vi "camera defaults globals - SubVI.vi"() -> ()   [LabVIEW 2014]
uses:
  Glimpse-master/Microscope plugins/Camera/Image size.ctt
panel:
  in  "Image Size Limits":T1={"H Bin"=1, "V Bin"=1, "Left"=1, "Top"=1, "Right"=512, "Bottom"=512}
  in  "Default Image Size":T1={"H Bin"=1, "V Bin"=1, "Left"=6, "Top"=1, "Right"=305, "Bottom"=512}
  # "ixon 512"
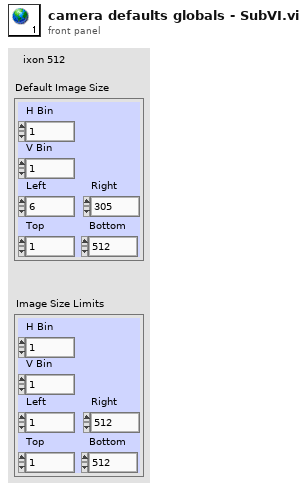
[diagram p1: front panel]
types:
  T1 = typedef "Image size.ctt" = cluster{"H Bin":i32, "V Bin":i32, "Left":i32, "Top":i32, "Right":i32, "Bottom":i32}
diagram:
